vi "Img_measure_lanes.vi"(7 "img_name":string, 8 "error in (no error)":errorcluster, 9 "Lanes":cluster{"X":dbl, "Y":dbl}[][](array[cluster]), 10 "BirdEyeView_params":T2, 11 "Image":T1(plugin-control)) -> (0 "error out":errorcluster, 2 "detected_points":cluster{"X":sgl, "Y":sgl}[][](array[cluster]), 3 "Image out":T1(plugin-control))   [LabVIEW 2021, in "Framework_lib.lvlib"]
uses:
  QMH/Framework_lib.lvlib
  <vilib>/vision/Measure.llb/Edge Options.ctl
  <vilib>/vision/Measure.llb/Edge Polarity.ctl
  <vilib>/vision/NI_Vision_Development_Module.lvlib
panel:
  out "Gradient Values":dbl[](array[numeric])
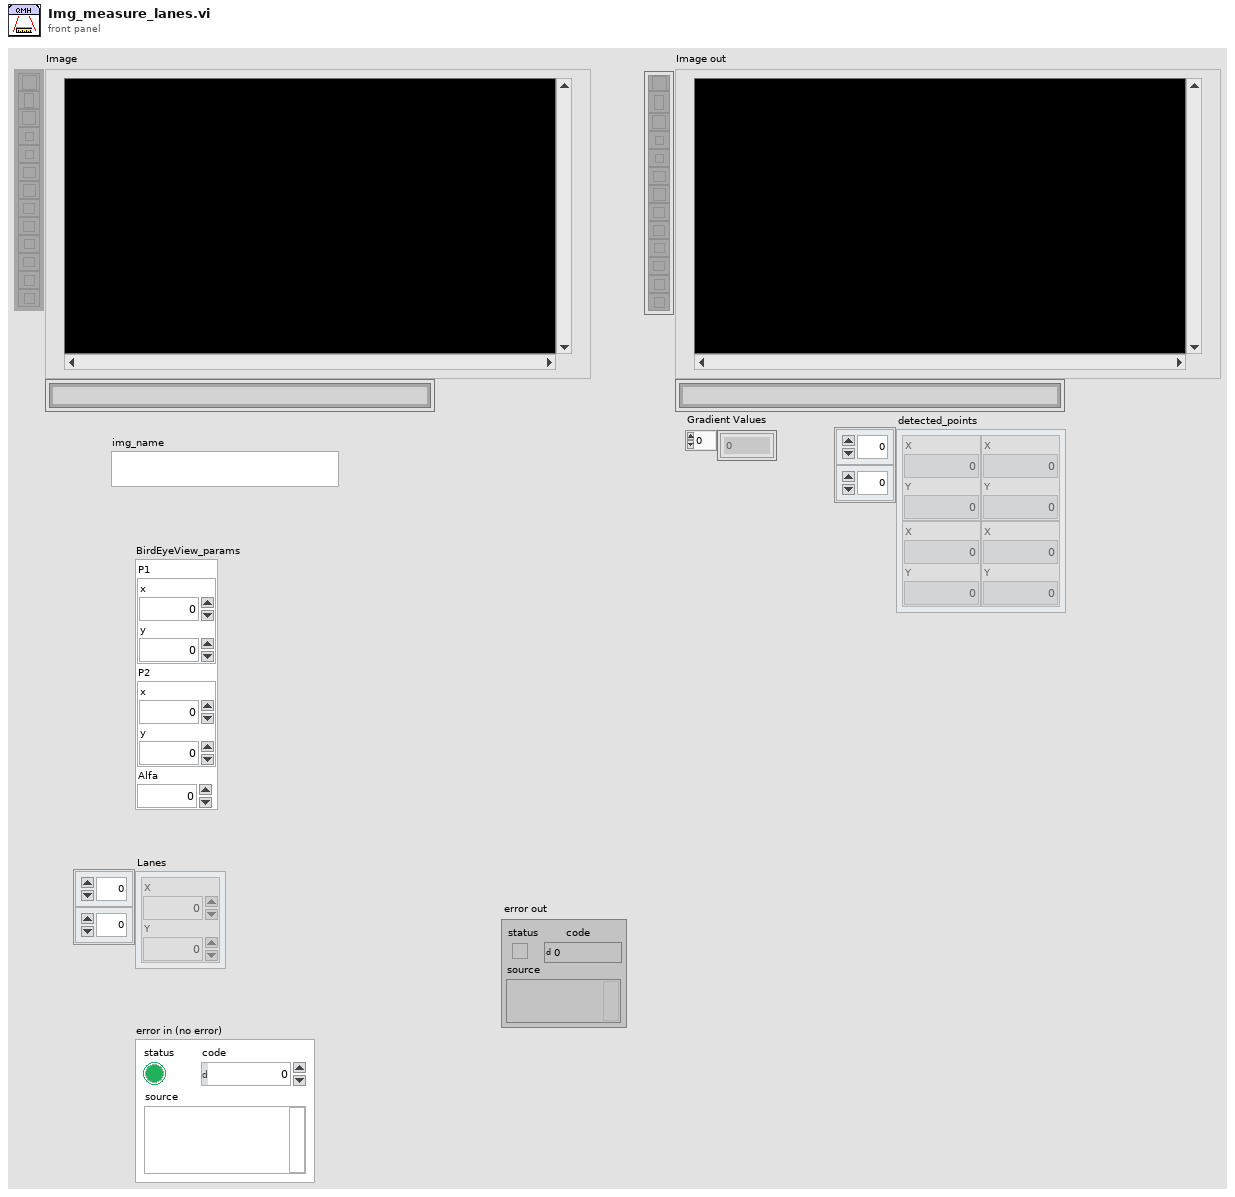
[diagram p1: front panel]
types:
  T1 = typedef "IMAQ Image.ctl" = refnum<image>
  T2 = cluster{"P1":cluster{"x":i16, "y":i16}, "P2":cluster{"x":i16, "y":i16}, "Alfa":dbl}
  T3 = typedef "ROI Descriptor" = cluster{"Global Rectangle":i32[], "Contours":cluster{"ID":enum32{"External", "Internal"}, "Type":u32, "Coordinates":i32[]}[]}
  T4 = typedef "Image Type" = u32
  T5 = typedef "Edge Options.ctl" = cluster{"Edge Polarity":T6, "Kernel Size":u32, "Width":u32, "Minimum Edge Strength":sgl, "Interpolation Type":enum32{"Zero Order", "Bilinear", "Quadratic", "Cubic", "Bilinear Fixed"}, "Data Processing Method":enum32{"Average", "Median"}}
  T6 = typedef "Edge Polarity.ctl" = u32
  T7 = enum16{"Get First Edge", "Get First + Last Edge", "Get All Edges", "Get Best Edge"}
  T8 = typedef "Edge New.ctl" = cluster{"Location (Pixel)":cluster{"X":sgl, "Y":sgl}, "Location (Real-World)":cluster{"X":sgl, "Y":sgl}, "Distance (Pixel)":dbl, "Distance (Real-World)":dbl, "Strength":dbl, "Noise":dbl, "Rising?":bool}
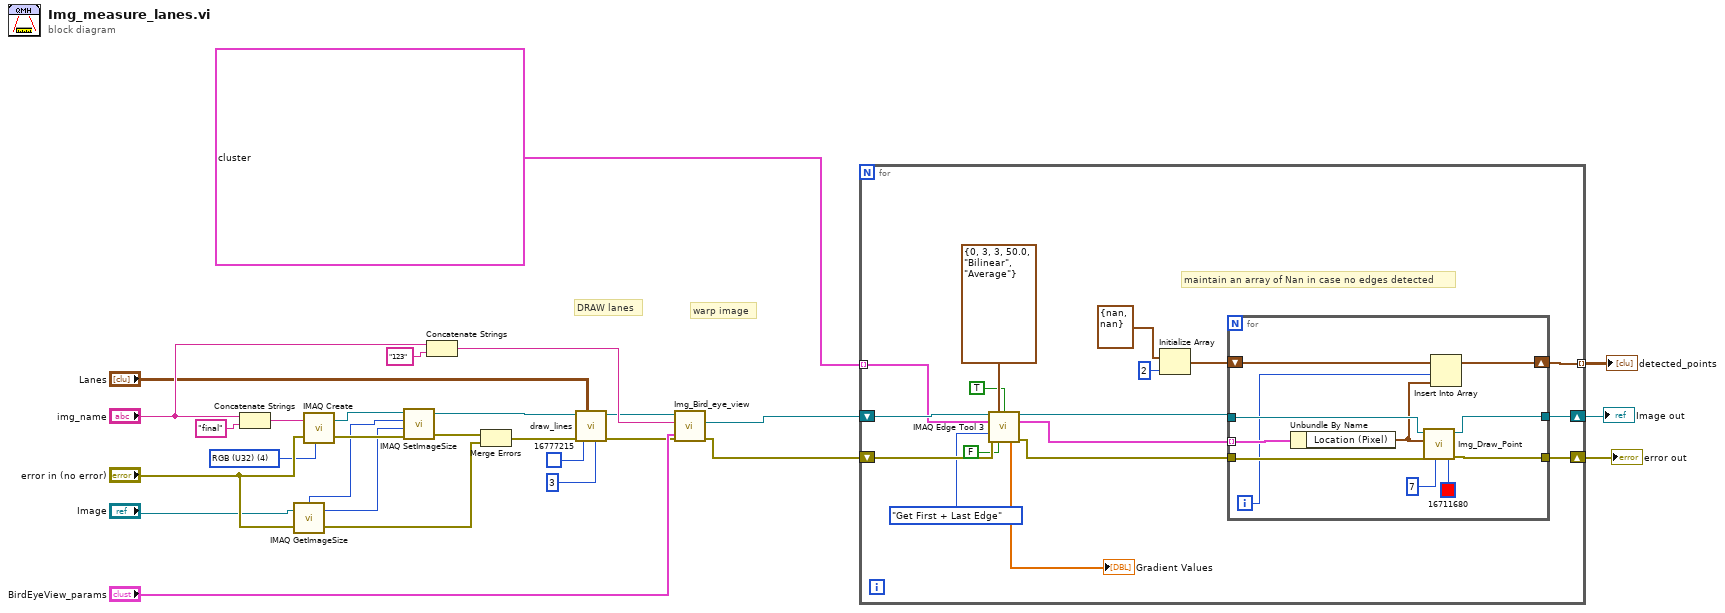
[diagram p0: block diagram]
diagram:
  w19 = T4 4 items=["Grayscale (U8)", "Grayscale (I16)", "Grayscale (SGL)", "Complex (CSG)", "RGB (U32)", "HSL (U32)", "RGB (U64)", "Grayscale (U16)"] ("Image Type")
  # "warp image"
  # "DRAW lanes"
  n1 = Concatenate Strings("img_name", "final" ("string")) -> (w24:string)
  n2 = call "IMAQ GetImageSize"("Image"="Image", "error in (no error)"="error in (no error)") -> ("Y Resolution"=w14:i32, "X Resolution"=w15:i32, "error out"=w12:errorcluster)  [unwired: 2 in]
  n3 = call "IMAQ Create"("Image Name"=w24, "Image Type"=w19, "error in (no error)"="error in (no error)") -> ("New Image"=w17:T1, "error out"=w16:errorcluster)  [unwired: 2 in]
  n4 = call "IMAQ SetImageSize"("error in (no error)"=w16, "Y Resolution"=w14, "X Resolution"=w15, "Image"=w17) -> ("error out"=w13:errorcluster, "Image Out"=w10:T1)  [unwired: 1 in]
  n5 = Concatenate Strings("img_name", "123" ("string")) -> (w28:string)
  n6 = Merge Errors(w13, w12) -> (w11:errorcluster)
  n7 = call "draw_lines.vi"("line_width"=3, "line_Color"=u32 16777215, "Lanes"="Lanes", "error in (no error)"=w11, "Image"=w10) -> ("error out"=w22:errorcluster, "Image out"=w23:T1)  [unwired: 5 in]
  n8 = call "Img_Bird_eye_view.vi"("parameters"="BirdEyeView_params", "error in (no error)"=w22, "Image Name"=w28, "img annotation in"=w23) -> ("error out"=w2:errorcluster, "img_corrected"=w9:T1)  [unwired: 5 in, 1 out]
  n9 = for {
    tunnel: T3[] [{"Global Rectangle"=[], "Contours"=[{"ID"=enum."External", "Type"=2, "Coordinates"=[383, 700, 1483, 700]}]}, {"Global Rectangle"=[], "Contours"=[{"ID"=enum."External", "Type"=2, "Coordinates"=[383, 1000, 1483, 1000]}]}] ("Array") -> [w34] mode=indexing
    shift-right: [w36] -> w5
    shift-left: w2 -> [w45]
    shift-right: [w37] -> w7
    shift-left: w9 -> [w43]
    tunnel: [w32] -> w3 mode=indexing
    # "maintain an array of Nan in case no edges detected"
    n10 = call "IMAQ Edge Tool 3"("Image"=w43, "Edge Options"=T5 {"Edge Polarity"=0, "Kernel Size"=3, "Width"=3, "Minimum Edge Strength"=50.0, "Interpolation Type"=enum."Bilinear", "Data Processing Method"=enum."Average"}, "Optimized Mode"=TRUE, "ROI Descriptor"=w34, "Process"=T7."Get First + Last Edge", "error in (no error)"=w45, "Reverse Direction"=FALSE) -> ("Image (duplicate)"=w39:T1, "Edge Information"=w33:T8[], "Gradient Values"=→"Gradient Values":dbl[], "error out"=w38:errorcluster)  [unwired: 4 in, 1 out]
    n11 = Initialize Array(cluster{"X":sgl, "Y":sgl} {"X"=nan, "Y"=nan} ("Location (Pixel)"), 2 ("dimension size")) -> (w30:cluster{"X":sgl, "Y":sgl}[])
    n12 = for {
      tunnel: w33 -> [w54] mode=indexing
      tunnel: w39 -> [w56]
      tunnel: w38 -> [w55]
      tunnel: [w53] -> w37
      tunnel: [w51] -> w36
      shift-right: [w50] -> w32
      shift-left: w30 -> [w49]
      i -> [w46]
      n13 = Unbundle By Name(w54) -> ("Location (Pixel)"=w48:cluster{"X":sgl, "Y":sgl})
      n14 = call "Img_Draw_Point.vi"("Color"=u32 16711680, "diameter"=u16 7, "error in (no error)"=w55, "Point Coordinates"=w48, "Image In"=w56) -> ("error out"=w51:errorcluster, "Image Out"=w53:T1)  [unwired: 5 in]
      n15 = Insert Into Array(array=w49, index=w46, new element=w48) -> (w50:cluster{"X":sgl, "Y":sgl}[])
    }
  }
  "Image out" <- w7
  "error out" <- w5
  "detected_points" <- w3
